vi "Get Diagnostics.vi"(8 "error in (no error)":errorcluster, 11 "Temperature Controller Driver in":refnum<class "Temperature Controller Driver.lvclass">) -> (0 "error out":errorcluster, 2 "Diagnostics":string, 3 "Temperature Controller Driver out":refnum<class "Temperature Controller Driver.lvclass">)   [LabVIEW 2024, in "Temperature Controller Driver.lvclass"]
uses:
  Temperature Controller Driver.lvclass
  Temperature Controller Driver.lvclass/Temperature Controller Driver.ctl
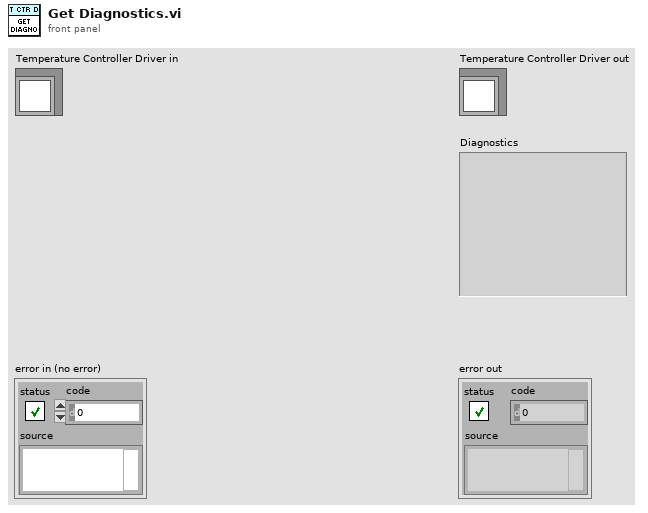
[diagram p1: front panel]
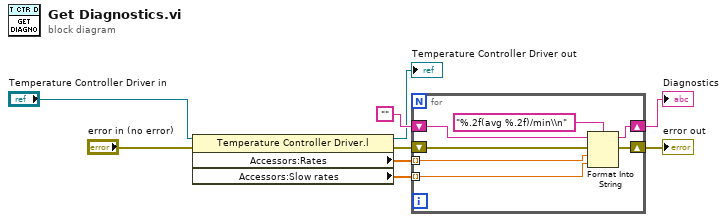
[diagram p0: block diagram]
diagram:
  n1 = property class="Temperature Controller Driver.l"(reference="Temperature Controller Driver in", error in="error in (no error)") -> (reference out=→"Temperature Controller Driver out":refnum<class "Temperature Controller Driver.lvclass">, error out=w7:errorcluster, "Accessors:Rates"=w6:dbl[], "Accessors:Slow rates"=w1:dbl[])
  n2 = for {
    tunnel: w6 -> [w13] mode=indexing
    shift-right: [w15] -> w3
    shift-left: w7 -> [w16]
    shift-right: [w11] -> w4
    shift-left: "" -> [w12]
    tunnel: w1 -> [w10] mode=indexing
    n3 = Format Into String(format string="%.2f(avg %.2f)/min\\n", initial string=w12, error in=w16, w13, w10) -> (resulting string=w11:string, error out=w15:errorcluster)
  }
  "error out" <- w3
  "Diagnostics" <- w4
